vi "I16 TO hex.vi"(11 "x":i16=-2137) -> (3 "concatenated string":string)   [LabVIEW 2017]
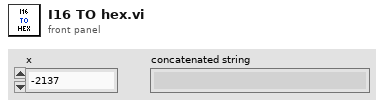
[diagram p1: front panel]
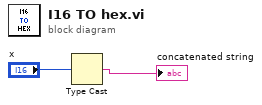
[diagram p0: block diagram]
diagram:
  n1 = Type Cast(x="x") -> (*(type *) &x=→"concatenated string":string)  [unwired: 1 in]
